vi "Update Plugin Selector.vi"(8 "error in (no error)":errorcluster, 11 "CIF_UI in":refnum<class "CIF_UI.lvclass">) -> (0 "error out":errorcluster)   [LabVIEW 2021, in "CIF_UI.lvclass"]
uses:
  CIF_UI.lvclass
  CIF_UI.lvclass/CIF_UI.ctl
  9cf455c6-64e3-46d3-bacc-62af7666256e.vi
  <vilib>/Comparison/Less/Less Functor/Less Functor.lvclass
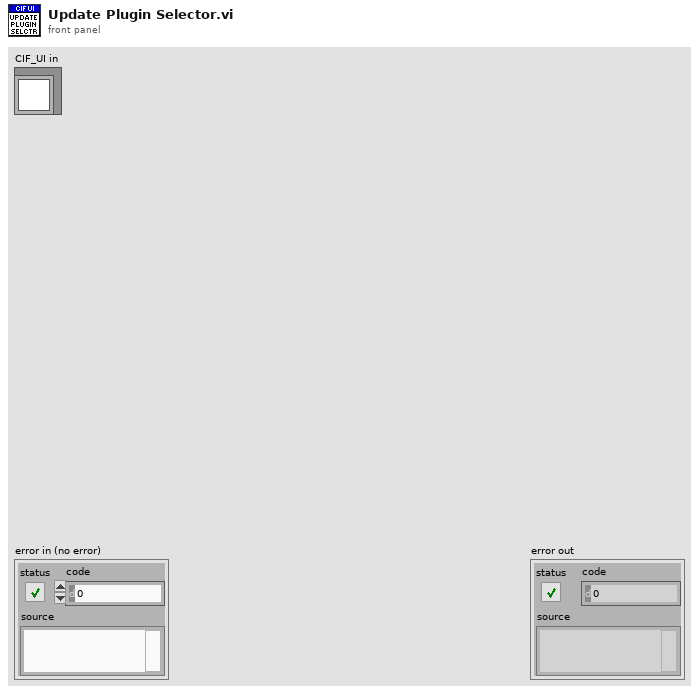
[diagram p1: front panel]
types:
  T1 = typedef "CIF_UI.lvclass/Plugin Connection Map.ctl" = map{string, T2}
  T2 = typedef "CIF_UI.lvclass/Plugin Connections.ctl" = cluster{"gRPC ID":T3, "Plugin Info":T4}
  T3 = typedef "grpc-lvsupport-release.lvlib/grpcId.ctl" = u64
  T4 = typedef "CIF_UI.lvclass/PluginInfo.ctl" = cluster{"Name":string, "Type":string, "grpc_port":i32, "Version":T5, "Node Status":T6}
  T5 = typedef "CIF_UI.lvclass/Version.ctl" = cluster{"Major":i32, "Minor":i32, "Fix":i32}
  T6 = typedef "CIFCoreCommon.lvlib/gRPC Reported Plugin Status.ctl" = cluster{"State":T7, "Timing Statistics (us)":T8, "FIFO Statistics (us)":T10, "error":T11, "Monitor Doubles":T12, "Monitor U64":T13, "Monitor I64":T14}
  T7 = typedef "CIFCoreCommon.lvlib/Plugin State.ctl" = enum32{"Null", "Creating", "Listening", "Running", "CleaningUp", "Destroying"}
  T8 = typedef "CIFCoreCommon.lvlib/Timing Statistics.ctl" = cluster{"Period":T9, "Wake Error":T9, "Execute":T9, "Housekeep":T9, "Idle":T9, "Cleanup":T9, "Custom 1 (custom units)":T9, "Custom 2 (custom units)":T9}
  T9 = typedef "CIFCoreCommon.lvlib/Timing Stats Base.ctl" = cluster{"Max":i64, "Avg":dbl, "Min":i64}
  T10 = typedef "CIFCoreCommon.lvlib/FIFO Statistics.ctl" = cluster{"From T0":T9, "From Previous Plugin":T9, "Output Error":T9}
  T11 = typedef "CIFCoreCommon.lvlib/Simple Error.ctl" = cluster{"status":bool, "code":i32}
  T12 = typedef "CIFCoreCommon.lvlib/Monitor Doubles.ctl" = cluster{"1":dbl, "2":dbl, "3":dbl, "4":dbl}
  T13 = typedef "CIFCoreCommon.lvlib/Monitor U64.ctl" = cluster{"1":u64, "2":u64, "3":u64, "4":u64}
  T14 = typedef "CIFCoreCommon.lvlib/Monitor I64.ctl" = cluster{"1":i64, "2":i64, "3":i64, "4":i64}
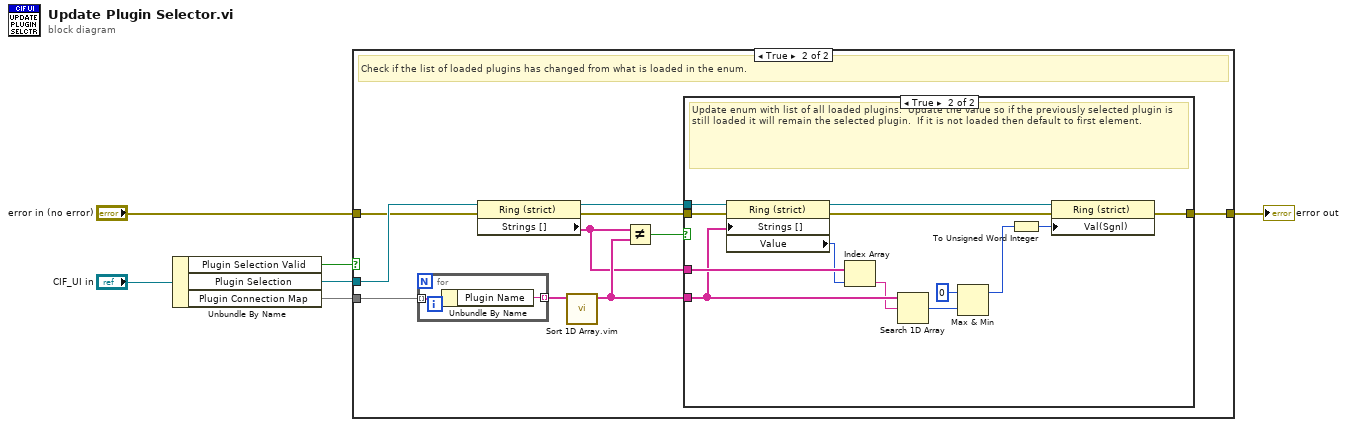
[diagram p0: block diagram]
diagram:
  n1 = Unbundle By Name("CIF_UI in") -> ("Plugin Selection Valid"=w5:bool, "Plugin Selection"=w3:refnum<vi>, "Plugin Connection Map"=w4:T1)
  n2 = case shown="True" w5 {
    tunnel: w4 -> [_ w17]
    tunnel: w3 -> [_ w15]
    tunnel: "error in (no error)" -> [w7 w10]
    tunnel: [w7 w9] -> w1
    frame False {
    }
    frame True {
      # "Check if the list of loaded plugins has changed from what is loaded in the enum."
      n3 = for {
        tunnel: w17 -> [w33] mode=indexing
        tunnel: [w32] -> w16 mode=indexing
        n4 = Unbundle By Name(w33) -> ("Plugin Name"=w32:string)
      }
      n5 = property class="Ring (strict)"(reference=w15, error in=w10) -> (reference out=w13:refnum<vi>, error out=w11:errorcluster, "Strings []"=w8:string[])
      n6 = call "Sort 1D Array.vim"("unsorted array"=w16) -> ("sorted array"=w12:string[])  [unwired: 10 in]
      n7 = Not Equal?(x=w8, y=w12) -> (x != y?=w14:bool)
      n8 = case shown="True" w14 {
        tunnel: w13 -> [_ w31]
        tunnel: w12 -> [_ w24]
        tunnel: w11 -> [w18 w30]
        tunnel: [w18 w27] -> w9
        tunnel: w8 -> [_ w26]
        frame False {
        }
        frame True {
          # "Update enum with list of all loaded plugins.  Update the value so if the previously selected plugin is still loaded it will remain the selected plugin.  If it is not loaded then default to first element."
          n9 = property class="Ring (strict)"(reference=w31, error in=w30, "Strings []"=w24) -> (reference out=w28:refnum<vi>, error out=w29:errorcluster, "Value"=w25:u16)
          n10 = Index Array(array=w26, index=w25) -> (element=w23:string)
          n11 = Search 1D Array(1D array=w24, element=w23) -> (index of element=w22:i32)  [unwired: 1 in]
          n12 = Max & Min(x=0, y=w22) -> (max(x,y)=w20:i32)  [unwired: 1 out]
          n13 = To Unsigned Word Integer(number=w20) -> (unsigned 16bit integer=w19:u16)
          n14 = property class="Ring (strict)"(reference=w28, error in=w29, "Val(Sgnl)"=w19) -> (error out=w27:errorcluster)  [unwired: 1 out]
        }
      }
    }
  }
  "error out" <- w1
